vi "RSZVB Query External Generator.vi"(0 "VISA session":refnum<visa-resource-name>, 5 "Generator Number (1)":i32=1, 11 "error in (no error)":errorcluster {"code" format="%.0x"}) -> (3 "Generator Name":string, 4 "dup VISA session":refnum<visa-resource-name>, 6 "Generator Type":string, 8 "Interface Type":string, 10 "Interface Address":string, 13 "10 MHz Reference Frequency":bool, 14 "Fast Sweep Mode":bool, 15 "error out":errorcluster {"code" format="%.0x"})   [LabVIEW 2011]
doc: "This VI queries an external generator.\n\nRemote-control command(s):\nSYSTem:COMMunicate:RDEVice:GENerator<gen_no>:DEFine?"
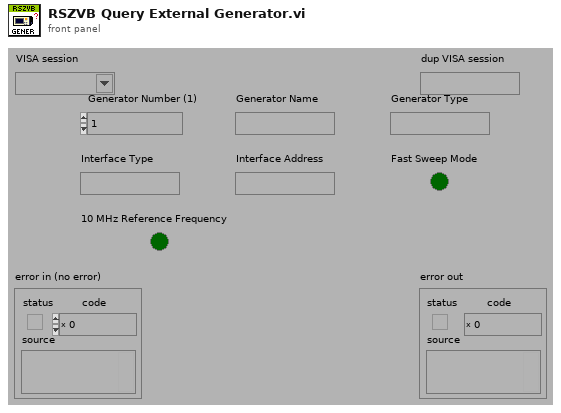
[diagram p1: front panel]
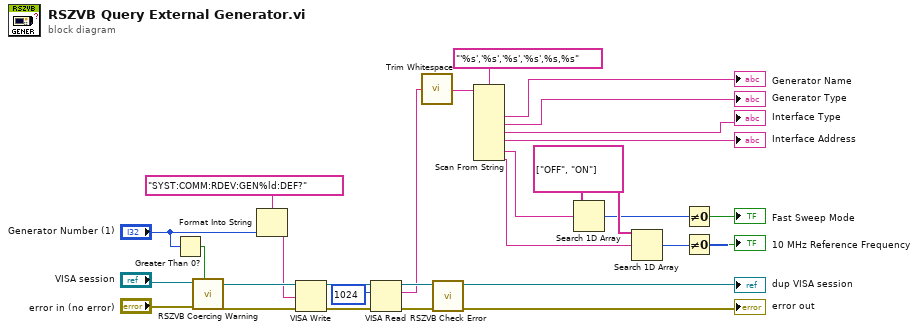
[diagram p0: block diagram]
diagram:
  w6 = string[] ["OFF", "ON"] ("array 2")
  n1 = Greater Than 0?(x="Generator Number (1)") -> (x > 0?=w20:bool)
  n2 = call "RSZVB Coercing Warning.vi"("In Range?"=w20, "error in (no error)"="error in (no error)", "VISA session"="VISA session") -> ("error out"=w22:errorcluster, "dup VISA session"=w21:refnum<visa-resource-name>)  [unwired: 7 in]
  n3 = Format Into String(format string="SYST:COMM:RDEV:GEN%ld:DEF?", "Generator Number (1)") -> (resulting string=w19:string)  [unwired: 2 in, 1 out]
  n4 = VISA Write(VISA resource name=w21, write buffer=w19, error in (no error)=w22) -> (VISA resource name out=w27:refnum<visa-resource-name>, error out=w29:errorcluster)  [unwired: 1 out]
  n5 = VISA Read(VISA resource name=w27, byte count=u32 1024 ("byte count (0)"), error in (no error)=w29) -> (VISA resource name out=w26:refnum<visa-resource-name>, read buffer=w24:string, error out=w25:errorcluster)  [unwired: 1 out]
  n6 = call <vilib>:"Trim Whitespace.vi"("string"=w24) -> ("trimmed string"=w17:string)  [unwired: 1 in]
  n7 = call "RSZVB Check Error.vi"("error in (no error)"=w25, "VISA session"=w26) -> ("error out"=→"error out":errorcluster, "dup VISA session"=→"dup VISA session":refnum<visa-resource-name>)  [unwired: 8 in]
  n8 = Scan From String(format string="'%s','%s','%s','%s',%s,%s", input string=w17) -> (output 1=→"Generator Name":string, output 2=→"Generator Type":string, output 3=→"Interface Type":string, output 4=→"Interface Address":string, output 5=w7:string, output 6=w5:string)  [unwired: 8 in, 3 out]
  n9 = Search 1D Array(1D array=w6, element=w7) -> (index of element=w3:i32)  [unwired: 1 in]
  n10 = Search 1D Array(1D array=w6, element=w5) -> (index of element=w4:i32)  [unwired: 1 in]
  n11 = Not Equal To 0?(x=w3) -> (x != 0?=→"Fast Sweep Mode":bool)
  n12 = Not Equal To 0?(x=w4) -> (x != 0?=→"10 MHz Reference Frequency":bool)
